vi "timeoutToShoot.vi"(8 "error in (no error)":errorcluster, 9 "timeoutToShoot":dbl, 10 "firstCallForState":bool=TRUE, 11 "KickToSkill in":refnum<class "KickToSkill.lvclass">) -> (0 "error out":errorcluster, 2 "elapsedTimeToShoot":bool, 3 "KickToSkill out":refnum<class "KickToSkill.lvclass">)   [LabVIEW 2021, in "KickToSkill.lvclass"]
uses:
  KickToSkill.lvclass
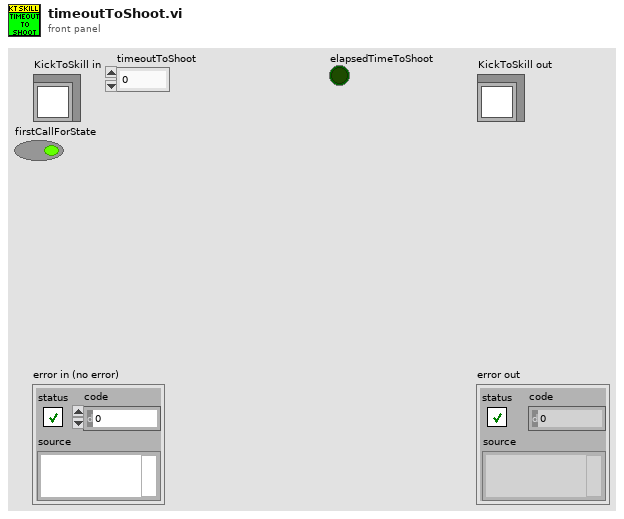
[diagram p1: front panel]
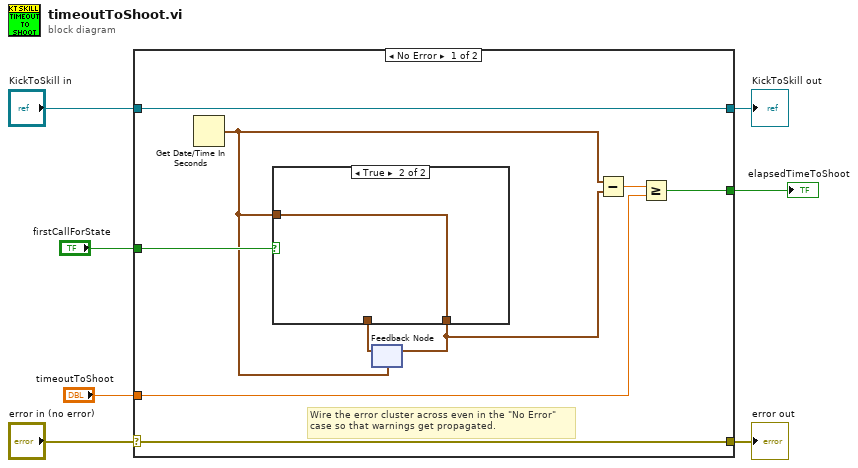
[diagram p0: block diagram]
diagram:
  n1 = case shown="No Error" "error in (no error)" {
    selector: "error in (no error)" -> [w15 w20]
    tunnel: [w15 w20] -> w6
    tunnel: [w16 w19] -> w4
    tunnel: "KickToSkill in" -> [w16 w19]
    tunnel: "firstCallForState" -> [w14 _]
    tunnel: "timeoutToShoot" -> [w9 _]
    tunnel: [w8 _] -> w1
    frame No Error {
      # "Wire the error cluster across even in the \"No Error\"\ncase so that warnings get propagated."
      n2 = Get Date/Time In Seconds() -> (seconds since 1Jan1904=w12:timestamp)
      n3 = feedback #1(w12) -> (w13:timestamp)
      n4 = case shown="True" w14 {
        tunnel: [w17 w18] -> w11
        tunnel: w12 -> [_ w18]
        tunnel: w13 -> [w17 _]
        frame False {
        }
        frame True {
        }
      }
      n5 = feedback-in #1(w11) -> ()
      n6 = Subtract(x=w12, y=w11) -> (x-y=w10:dbl)
      n7 = Greater Or Equal?(x=w10, y=w9) -> (x >= y?=w8:bool)
    }
    frame Error {
    }
  }
  "error out" <- w6
  "KickToSkill out" <- w4
  "elapsedTimeToShoot" <- w1
